vi "Active Drive Test Sync.vi"() -> ()   [LabVIEW 2015]
uses:
  <vilib>/DAQmx/write.llb/DAQmx Write (Digital Bool 1Line 1Point).vi
  <vilib>/DAQmx/create/channels.llb/DAQmx Create Channel (DO-Digital Output).vi
  <vilib>/DAQmx/miscellaneous.llb/DAQmx Fill In Error Info.vi
  <resource>/objmgr/daqmx.rc
panel:
  in  "Stop Button":bool
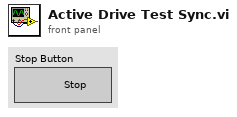
[diagram p1: front panel]
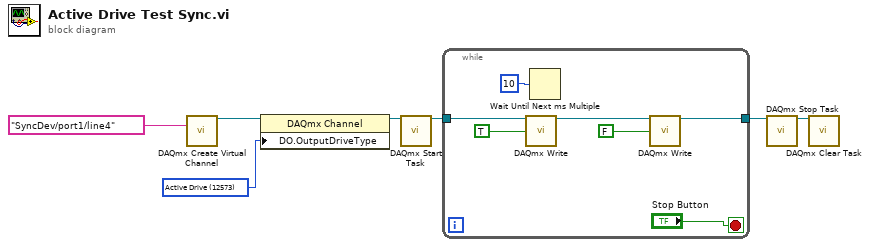
[diagram p0: block diagram]
diagram:
  w7 = 12573 items=["Active Drive"=12573, "Open Collector"=12574] ("DO.OutputDriveType")
  n1 = call-poly <vilib>:"DAQmx Create Virtual Channel.vi"("lines"=tag "SyncDev/port1/line4") -> ("task out"=w2:refnum<k21>)  [unwired: 13 in, 1 out]
  n2 = property class="DAQmx Channel"(reference=w2, "DO.OutputDriveType"=w7) -> (reference out=w1:refnum<k21>)  [unwired: 1 in, 1 out]
  n3 = call <vilib>:"DAQmx Start Task.vi"("task/channels in"=w1) -> ("task out"=w4:refnum<k21>)  [unwired: 13 in, 1 out]
  n4 = while {
    tunnel: w4 -> [w14]
    tunnel: [w9] -> w5
    stop <- "Stop Button" stop-if-true
    n5 = call-poly <vilib>:"DAQmx Write.vi"("task/channels in"=w14, "data"=TRUE) -> ("task out"=w13:refnum<k21>)  [unwired: 11 in, 2 out]
    n6 = Wait Until Next ms Multiple(millisecond multiple=u32 10) -> ()  [unwired: 1 out]
    n7 = call-poly <vilib>:"DAQmx Write.vi"("task/channels in"=w13, "data"=FALSE) -> ("task out"=w9:refnum<k21>)  [unwired: 11 in, 2 out]
  }
  n8 = call <vilib>:"DAQmx Stop Task.vi"("task/channels in"=w5) -> ("task out"=w6:refnum<k21>)  [unwired: 13 in, 1 out]
  n9 = call <vilib>:"DAQmx Clear Task.vi"("task in"=w6) -> ()  [unwired: 14 in, 1 out]
